vi "WhileLoopDemo2.vi"() -> ()   [LabVIEW 2018]
panel:
  out "Triggered":bool
  in  "Threshold":dbl
  in  "Slide":dbl(slide) scale=0.0..10.0
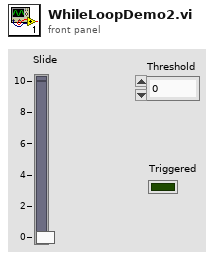
[diagram p1: front panel]
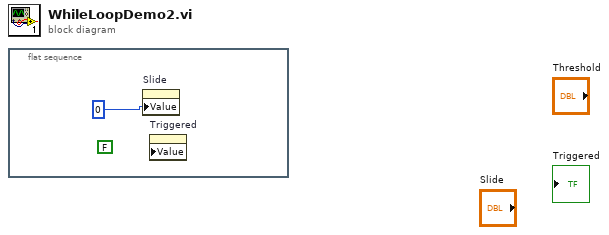
[diagram p0: block diagram]
diagram:
  n1 = flat-sequence {
    frame #0 {
      (unwired) FALSE
      n2 = property on="Slide" class="Slide (strict)"("Value"=0) -> ()  [unwired: 2 in, 2 out]
      n3 = property on="Triggered" class="Bool (strict)" props=["Value"]() -> ()  [unwired: 3 in, 2 out]
    }
  }
